vi "LeerBaseDatos_externo.vi"(8 "error in (no error)":errorcluster, 11 "Prueba01 in":refnum<class "Prueba01.lvclass">) -> (0 "error out":errorcluster, 3 "Prueba01 out":refnum<class "Prueba01.lvclass">)   [LabVIEW 2019, in "Prueba01.lvclass"]
uses:
  Prueba01.lvclass
  Controles/BD_P01.ctl
  Prueba01.lvclass/Prueba01.ctl
  Base de Datos/SQLiteConnector/SQLiteConnection.lvclass
  Base de Datos/Base de Datos.lvclass
panel:
  out "NPS Ref segun Fre_Ref":string
  out "BD":T1
  in  "Tipo Equipo":enum16{"Sonometro", "Calibrador", "Dosimetro"}(ring)
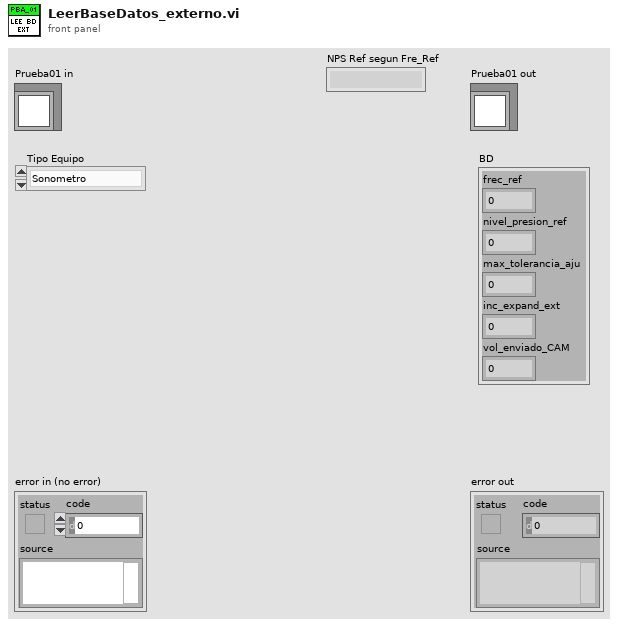
[diagram p1: front panel]
types:
  T1 = typedef "Prueba01.lvclass/BD_P01.ctl" = cluster{"frec_ref":dbl, "nivel_presion_ref":dbl, "max_tolerancia_aju":dbl, "inc_expand_ext":dbl, "vol_enviado_CAM":dbl}
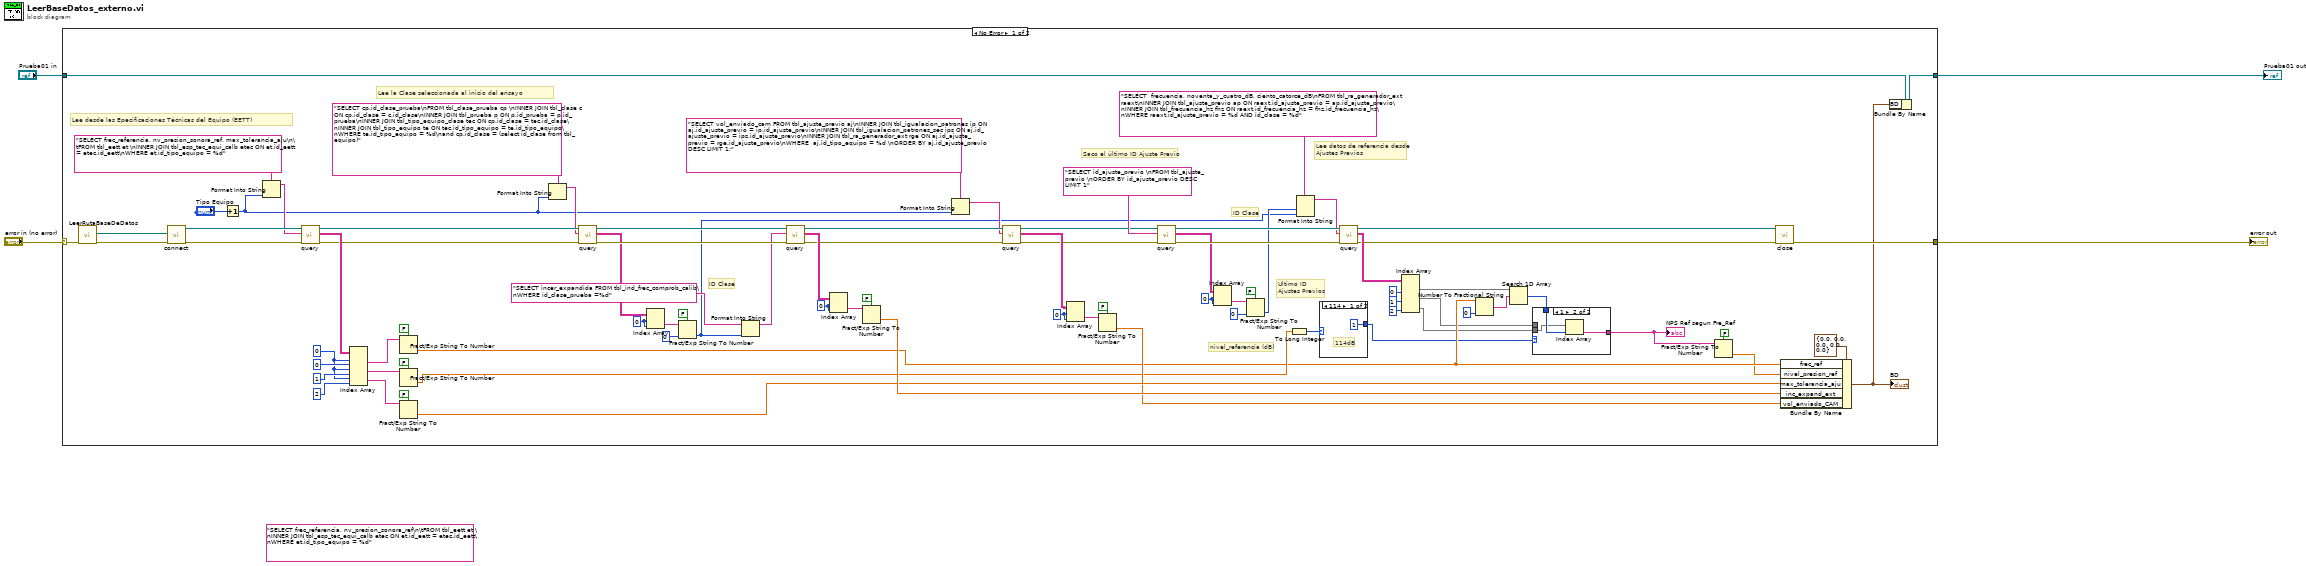
[diagram p0: block diagram]
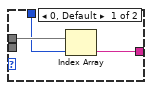
[diagram p2: hidden frame]
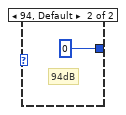
[diagram p3: hidden frame]
diagram:
  (unwired) "SELECT frec_referencia, nv_presion_sonora_ref\n\tFROM tbl_eett et \nINNER JOIN tbl_esp_tec_equi_calb etec ON et.id_eett = etec.id_eett\nWHERE et.id_tipo_equipo = %d" ("format string")
  n1 = case shown="No Error" "error in (no error)" {
    selector: "error in (no error)" -> [w89 w100]
    tunnel: [w81 w100] -> w3
    tunnel: [w49 w99] -> w1
    tunnel: "Prueba01 in" -> [w90 w99]
    frame No Error {
      w30 = 0 ("index (row)")
      w42 = 0 ("index (row)")
      w54 = 0 ("index (row)")
      w64 = 0 ("index (row)")
      w73 = 0 ("index (row)")
      # "ID Clase"
      # "Lee desde las Epecificaciones Técnicas del Equipo (EETT)"
      # "Lee la Clase seleccionada al inicio del ensayo"
      # "Ultimo ID\nAjustes Previos"
      # "ID Clase"
      # "Lee datos de referencia desde\nAjustes Previos"
      # "Saco el último ID Ajuste Previo"
      # "nivel_referencia (dB)"
      n2 = call "LeerRutaBaseDeDatos.vi"("error in (no error)"=w89) -> ("error out"=w83:errorcluster, "Database Path"=w82:path)  [unwired: 9 in]
      n3 = call "connect.vi"("error in (no error)"=w83, "Database Path"=w82) -> ("error out"=w85:errorcluster, "object out"=w86:refnum<class "SQLiteConnection.lvclass">)  [unwired: 8 in]
      n4 = Increment(x="Tipo Equipo") -> (x+1=w43:enum16{"Sonometro", "Calibrador", "Dosimetro"})
      n5 = Format Into String(format string="SELECT frec_referencia, nv_presion_sonora_ref, max_tolerancia_aju\n\tFROM tbl_eett et \nINNER JOIN tbl_esp_tec_equi_calb etec ON et.id_eett = etec.id_eett\nWHERE et.id_tipo_equipo = %d", w43) -> (resulting string=w84:string)  [unwired: 2 in, 1 out]
      n6 = call "query.vi"("error in (no error)"=w85, "SQL Statement"=w84, "object in"=w86) -> ("error out"=w69:errorcluster, "result"=w80:string[][], "object out"=w68:refnum<class "SQLiteConnection.lvclass">)  [unwired: 5 in, 1 out]
      n7 = Index Array(array=w80, index (row) #1=w73, index (col) #1=0 ("disabled index (col)"), index (row) #2=w73, index (col) #2=1 ("disabled index (col)"), index (row) #3=w73, index (col) #3=2 ("index (col)")) -> (element #1=w77:string, element #2=w76:string, element #3=w71:string)
      n8 = Fract/Exp String To Number(use system decimal point (T)=FALSE, string=w77) -> (number=w16:dbl)  [unwired: 2 in, 1 out]
      n9 = Fract/Exp String To Number(use system decimal point (T)=FALSE, string=w76) -> (number=w19:dbl)  [unwired: 2 in, 1 out]
      n10 = Fract/Exp String To Number(use system decimal point (T)=FALSE, string=w71) -> (number=w50:dbl)  [unwired: 2 in, 1 out]
      n11 = Format Into String(format string="SELECT cp.id_clase_prueba\nFROM tbl_clase_prueba cp \nINNER JOIN tbl_clase c ON cp.id_clase = c.id_clase\nINNER JOIN tbl_prueba p ON p.id_prueba = p.id_prueba\nINNER JOIN tbl_tipo_equipo_clase tec ON cp.id_clase = tec.id_clase\nINNER JOIN tbl_tipo_equipo te ON tec.id_tipo_equipo = te.id_tipo_equipo\nWHERE te.id_tipo_equipo = %d\nand cp.id_clase = (select id_clase from tbl_equipo)", w43) -> (resulting string=w66:string)  [unwired: 2 in, 1 out]
      n12 = call "query.vi"("error in (no error)"=w69, "SQL Statement"=w66, "object in"=w68) -> ("error out"=w65:errorcluster, "result"=w63:string[][], "object out"=w57:refnum<class "SQLiteConnection.lvclass">)  [unwired: 5 in, 1 out]
      n13 = Index Array(array=w63, index (row)=w64, index (col)=w64) -> (element=w61:string)
      n14 = Fract/Exp String To Number(use system decimal point (T)=FALSE, string=w61, default (0 dbl)=0 ("index (row)")) -> (number=w21:i32)  [unwired: 1 in, 1 out]
      n15 = Format Into String(format string="SELECT incer_expandida FROM tbl_ind_frec_comprob_calib\nWHERE id_clase_prueba =%d", w21) -> (resulting string=w58:string)  [unwired: 2 in, 1 out]
      n16 = call "query.vi"("error in (no error)"=w65, "SQL Statement"=w58, "object in"=w57) -> ("error out"=w46:errorcluster, "result"=w53:string[][], "object out"=w47:refnum<class "SQLiteConnection.lvclass">)  [unwired: 5 in, 1 out]
      n17 = Index Array(array=w53, index (row)=w54, index (col)=w54) -> (element=w56:string)
      n18 = Fract/Exp String To Number(use system decimal point (T)=FALSE, string=w56) -> (number=w51:dbl)  [unwired: 2 in, 1 out]
      n19 = Format Into String(format string="SELECT vol_enviado_cam FROM tbl_ajuste_previo aj\nINNER JOIN tbl_igualacion_patrones ip ON aj.id_ajuste_previo = ip.id_ajuste_previo\nINNER JOIN tbl_igualacion_patrones_sec ips ON aj.id_ajuste_previo = ips.id_ajuste_previo\nINNER JOIN tbl_ra_generador_ext rge ON aj.id_ajuste_previo = rge.id_ajuste_previo\nWHERE  aj.id_tipo_equipo = %d \nORDER BY aj.id_ajuste_previo DESC LIMIT 1;", w43) -> (resulting string=w44:string)  [unwired: 2 in, 1 out]
      n20 = call "query.vi"("error in (no error)"=w46, "SQL Statement"=w44, "object in"=w47) -> ("error out"=w23:errorcluster, "result"=w39:string[][], "object out"=w22:refnum<class "SQLiteConnection.lvclass">)  [unwired: 5 in, 1 out]
      n21 = Index Array(array=w39, index (row)=w42, index (col)=w42) -> (element=w40:string)
      n22 = Fract/Exp String To Number(use system decimal point (T)=FALSE, string=w40) -> (number=w38:dbl)  [unwired: 2 in, 1 out]
      n23 = call "query.vi"("error in (no error)"=w23, "SQL Statement"="SELECT id_ajuste_previo \nFROM tbl_ajuste_previo \nORDER BY id_ajuste_previo DESC LIMIT 1" ("format string"), "object in"=w22) -> ("error out"=w36:errorcluster, "result"=w29:string[][], "object out"=w35:refnum<class "SQLiteConnection.lvclass">)  [unwired: 5 in, 1 out]
      n24 = Index Array(array=w29, index (row)=w30, index (col)=w30) -> (element=w32:string)
      n25 = Fract/Exp String To Number(use system decimal point (T)=FALSE, string=w32, default (0 dbl)=0 ("index (row)")) -> (number=w24:i32)  [unwired: 1 in, 1 out]
      n26 = To Long Integer(number=w19) -> (32bit integer=w20:i32)
      n27 = Format Into String(format string="SELECT  frecuencia, noventa_y_cuatro_dB, ciento_catorce_dB\nFROM tbl_ra_generador_ext raext\nINNER JOIN tbl_ajuste_previo ap ON raext.id_ajuste_previo = ap.id_ajuste_previo\nINNER JOIN tbl_frecuencia_hz fhz ON raext.id_frecuencia_hz = fhz.id_frecuencia_hz\nWHERE raext.id_ajuste_previo = %d AND id_clase = %d", w24, w21) -> (resulting string=w27:string)  [unwired: 2 in, 1 out]
      n28 = case shown="114" w20 {
        tunnel: [1 ("disabled index (col)") 0 ("disabled index (col)")] -> w11
        frame 114 {
          # "114dB"
        }
        frame 94, Default {
          # "94dB"
        }
      }
      n29 = call "query.vi"("error in (no error)"=w36, "SQL Statement"=w27, "object in"=w35) -> ("error out"=w8:errorcluster, "result"=w37:string[][], "object out"=w9:refnum<class "SQLiteConnection.lvclass">)  [unwired: 5 in, 1 out]
      n30 = Index Array(array=w37, index (col) #1=0 ("disabled index (col)"), index (col) #2=1 ("index (col)"), index (col) #3=2 ("index (col)")) -> (element #1=w18:string[], element #2=w13:string[], element #3=w10:string[])  [unwired: 3 in]
      n31 = Number To Fractional String(number=w16, precision (6)=i16 0) -> (F-format string=w17:string)  [unwired: 2 in]
      n32 = Search 1D Array(1D array=w18, element=w17) -> (index of element=w12:i32)  [unwired: 1 in]
      n33 = case shown="1" w11 {
        tunnel: w13 -> [w93 _]
        tunnel: w12 -> [w92 w96]
        tunnel: w10 -> [_ w95]
        tunnel: [w91 w94] -> w7
        frame 0, Default {
          n34 = Index Array(array=w93, index=w92) -> (element=w91:string)
        }
        frame 1 {
          n35 = Index Array(array=w95, index=w96) -> (element=w94:string)
        }
      }
      "NPS Ref segun Fre_Ref" <- w7
      n36 = Fract/Exp String To Number(use system decimal point (T)=FALSE, string=w7) -> (number=w6:dbl)  [unwired: 2 in, 1 out]
      n37 = call-dynamic "close.vi"("error in (no error)"=w8, "object in"=w9) -> ("error out"=w81:errorcluster)  [unwired: 8 in, 1 out]
      n38 = Bundle By Name(cluster=T1 {"frec_ref"=0.0, "nivel_presion_ref"=0.0, "max_tolerancia_aju"=0.0, "inc_expand_ext"=0.0, "vol_enviado_CAM"=0.0}, "frec_ref"=w16, "nivel_presion_ref"=w6, "max_tolerancia_aju"=w50, "inc_expand_ext"=w51, "vol_enviado_CAM"=w38) -> (w48:T1)
      "BD" <- w48
      n39 = Bundle By Name(cluster=w90, "BD"=w48) -> (w49:refnum<class "Prueba01.lvclass">)
    }
    frame Error {
    }
  }
  "error out" <- w3
  "Prueba01 out" <- w1
